vi "EXT.vi"(5 "format string (%.;%#_20f)":string="%.;%#_20f", 7 "key description":string, 8 "sections":string[](array[string]), 9 "numeric":ext, 11 "info data":string) -> (0 "sections out":string[](array[string]), 3 "info data out":string)   [LabVIEW 2020, in "infolib.lvlib"]
doc: "Add a new numeric key to Info Data string. If section exists in Info Data string, inserts key into this section."
uses:
  infolib.lvlib
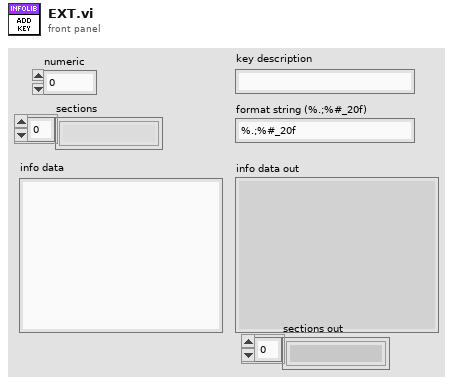
[diagram p1: front panel]
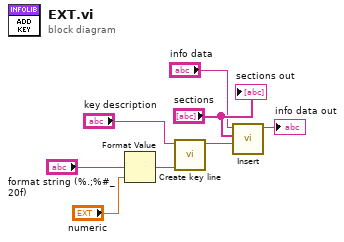
[diagram p0: block diagram]
diagram:
  n1 = Format Value(format string="format string (%.;%#_20f)", value (0)="numeric") -> (output string=w2:string)  [unwired: 1 in]
  n2 = call "Create key line.vi"("formatted value"=w2, "key description"="key description") -> ("line"=w1:string)  [unwired: 9 in]
  n3 = call "Insert.vi"("insert"=w1, "sections"="sections", "info data"="info data") -> ("info data out"=→"info data out":string)  [unwired: 8 in]
  "sections out" <- "sections"
